vi "Get as DBL.vi"(8 "error in (no error)":errorcluster, 10 "Name Array":string[](array[string]), 11 "JSON Value in":refnum<class "JSON Value.lvclass">) -> (0 "error out":errorcluster, 2 "Number":dbl, 3 "JSON Value out":refnum<class "JSON Value.lvclass">)   [LabVIEW 2020, in "Library Commun.lvlib" / "JSON Scalar.lvclass"]
doc: "Converts a <b>JSON Value</b> into a <b>Number</b>.\n\nCopyright 2012 James David Powell, Shaun Rumbell and Ton Plomp\nMore information on http://lavag.org/topic/16217-cr-json-labview"
uses:
  JSON Scalar.lvclass
  JSON Value/JSON Value.lvclass
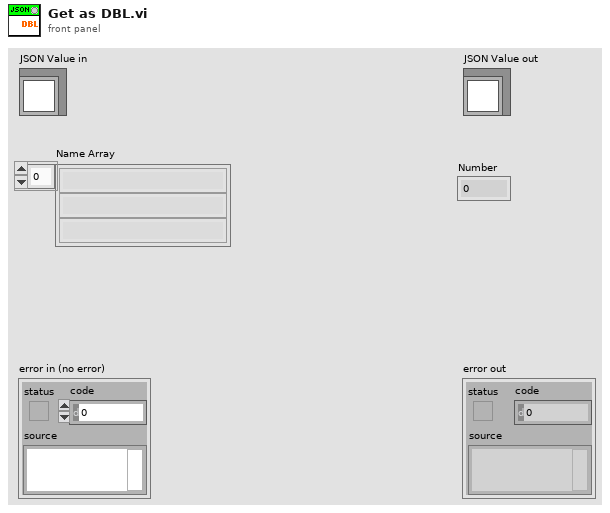
[diagram p1: front panel]
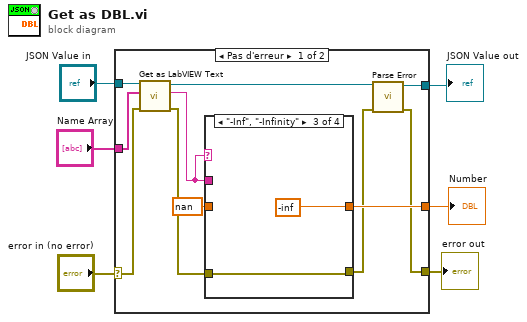
[diagram p0: block diagram]
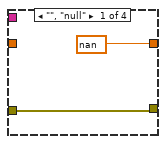
[diagram p2: hidden frame]
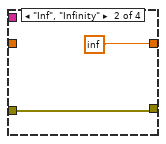
[diagram p3: hidden frame]
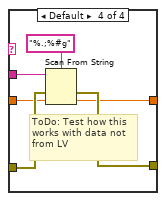
[diagram p4: hidden frame]
diagram:
  n1 = case shown="Pas d'erreur" "error in (no error)" {
    selector: "error in (no error)" -> [w8 w31]
    tunnel: [w17 _] -> w6
    tunnel: "JSON Value in" -> [w15 w30]
    tunnel: [w12 w30] -> w4
    tunnel: [w11 w31] -> w3
    tunnel: "Name Array" -> [w7 _]
    frame No Error {
      n2 = call-dynamic "Get as LabVIEW Text.vi"("error in (no error)"=w8, "Name Array"=w7, "JSON Value In"=w15) -> ("error out"=w9:errorcluster, "LabVIEW Text"=w14:string, "JSON Value Out"=w13:refnum<class "JSON Value.lvclass">)  [unwired: 5 in, 1 out]
      n3 = case shown="\"-Inf\", \"-Infinity\"" w14 {
        tunnel: [nan ("default value 1") inf ("default value 1") -inf ("default value 1") w25] -> w17
        tunnel: w9 -> [w18 w20 w22 w29]
        tunnel: [w18 w20 w22 w28] -> w10
        tunnel: nan ("default value 1") -> [_ _ _ w27]
        tunnel: w14 -> [_ _ _ w26]
        frame "", "null" {
        }
        frame "Inf", "Infinity" {
        }
        frame "-Inf", "-Infinity" {
        }
        frame Default {
          # "ToDo: Test how this\nworks with data not\nfrom LV"
          n4 = Scan From String(format string="%.;%#g", input string=w26, error in=w29, default 1=w27) -> (error out=w28:errorcluster, output 1=w25:dbl)  [unwired: 1 in, 2 out]
        }
      }
      n5 = call-dynamic "Parse Error.vi"("error in (no error)"=w10, "JSON Value in"=w13) -> ("error out"=w11:errorcluster, "JSON Value out"=w12:refnum<class "JSON Value.lvclass">)  [unwired: 8 in]
    }
    frame Error {
    }
  }
  "error out" <- w3
  "JSON Value out" <- w4
  "Number" <- w6
